vi "ParseArgumentsCore.vi"(8 "error in (no error)":errorcluster, 10 "Inputs":string[](array[string]), 11 "VIPMInstallPackageFile in":refnum<class "VIPMInstallPackageFile.lvclass">) -> (0 "error out":errorcluster, 3 "VIPMInstallPackageFile out":refnum<class "VIPMInstallPackageFile.lvclass">)   [LabVIEW 2014, in "VIPMInstallPackageFile.lvclass"]
uses:
  <nishared>/LabVIEW CLI/Operations/VIPMInstallPackageFile/VIPMInstallPackageFile.lvclass
  <nishared>/LabVIEW CLI/Operations/Utilities/OperationErrorType.ctl
  <nishared>/LabVIEW CLI/Operations/VIPMInstallPackageFile/VIPMInstallPackageFile.lvclass/VIPMInstallPackageFile.ctl
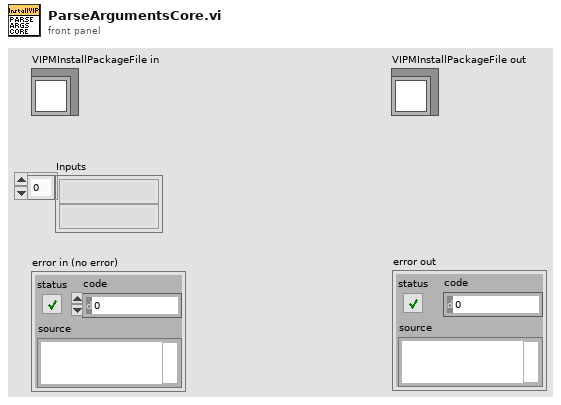
[diagram p1: front panel]
types:
  T1 = typedef "OperationErrorType.ctl" = enum16{"RequiredArgumentMissing", "UnknownArguments", "LoggerSetMultipleTimes", "OperationBrokenError"}
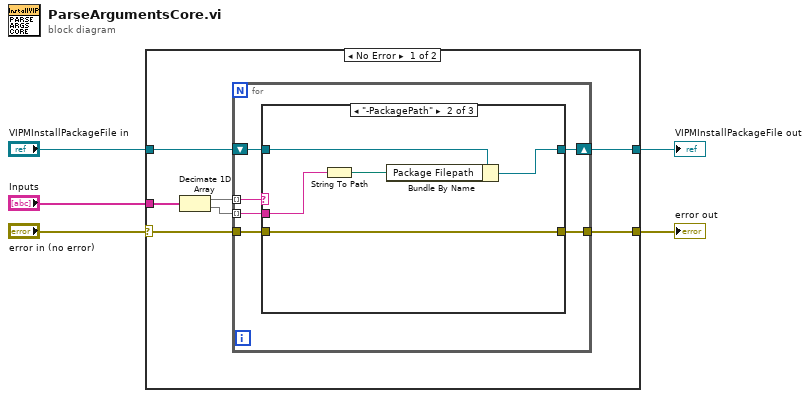
[diagram p0: block diagram]
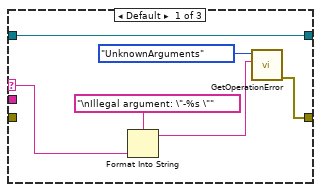
[diagram p2: hidden frame]
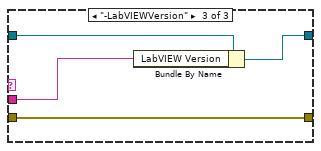
[diagram p3: hidden frame]
diagram:
  n1 = case shown="No Error" "error in (no error)" {
    selector: "error in (no error)" -> [w6 w35]
    tunnel: [w12 w35] -> w5
    tunnel: "Inputs" -> [w9 _]
    tunnel: "VIPMInstallPackageFile in" -> [w8 w34]
    tunnel: [w7 w34] -> w2
    frame No Error {
      n2 = Decimate 1D Array(w9) -> (w10:string[], w11:string[])
      n3 = for {
        tunnel: w10 -> [w18] mode=indexing
        tunnel: w11 -> [w17] mode=indexing
        shift-right: [w15] -> w7
        shift-left: w8 -> [w16]
        tunnel: w6 -> [w14]
        tunnel: [w13] -> w12
        n4 = case shown="\"-PackagePath\"" w18 {
          selector: w18 -> [w21 _ _]
          tunnel: w17 -> [_ w28 w32]
          tunnel: w16 -> [w24 w29 w33]
          tunnel: [w24 w26 w31] -> w15
          tunnel: w14 -> [_ w25 w30]
          tunnel: [w23 w25 w30] -> w13
          frame Default {
            n5 = Format Into String(format string="\nIllegal argument: \"-%s \"", w21) -> (resulting string=w19:string)  [unwired: 2 in, 1 out]
            n6 = call <nishared>:"GetOperationError.vi"("Additional Information"=w19, "Operation Error Type"=OperationErrorType."UnknownArguments") -> ("error out"=w23:errorcluster)  [unwired: 9 in]
          }
          frame "-PackagePath" {
            n7 = String To Path(string=w28) -> (path=w27:path)
            n8 = Bundle By Name(cluster=w29, "Package Filepath"=w27) -> (w26:refnum<class "VIPMInstallPackageFile.lvclass">)
          }
          frame "-LabVIEWVersion" {
            n9 = Bundle By Name(cluster=w33, "LabVIEW Version"=w32) -> (w31:refnum<class "VIPMInstallPackageFile.lvclass">)
          }
        }
      }
    }
    frame Error {
    }
  }
  "error out" <- w5
  "VIPMInstallPackageFile out" <- w2
